vi "ESP_WIFI_mod2 (1).vi"() -> ()   [LabVIEW 2020]
uses:
  <vilib>/httpClient/LabVIEWHTTPClient.lvlib
panel:
  in  "ESP32 IP":string
  in  "stop":bool
  in  "Port":u16
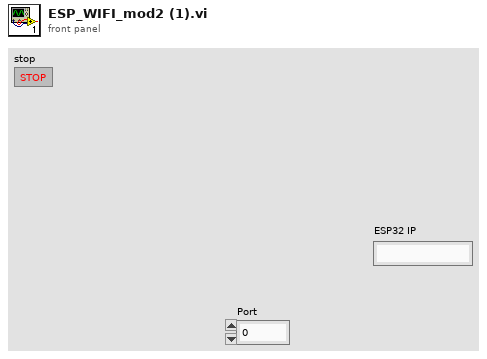
[diagram p1: front panel]
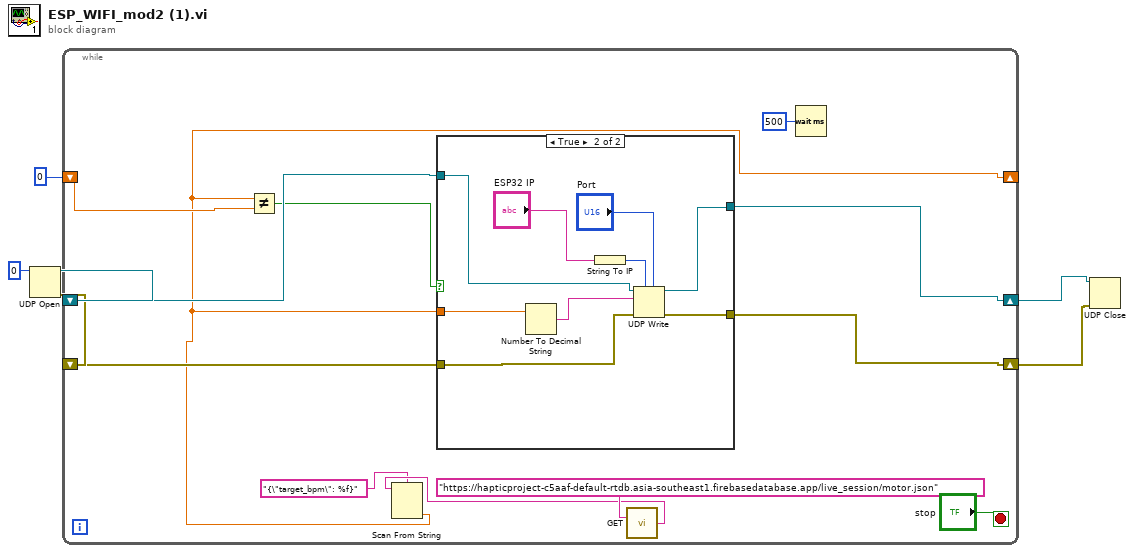
[diagram p0: block diagram]
diagram:
  n1 = UDP Open(11:u16 0 ("port")) -> (port=w6:refnum<k16>, 0:w5:errorcluster)  [unwired: 4 in, 1 out]
  n2 = while {
    shift-right: [w15] -> w4
    shift-left: w6 -> [w16]
    shift-right: [w13] -> w3
    shift-left: w5 -> [w14]
    shift-right: [w7] -> _
    shift-left: u16 0 ("port") -> [w9]
    stop <- "stop" stop-if-true
    n3 = call <vilib>:"GET.vi"("url"="https://hapticproject-c5aaf-default-rtdb.asia-southeast1.firebasedatabase.app/live_session/motor.json") -> ("body"=w11:string)  [unwired: 11 in, 3 out]
    n4 = Scan From String(format string="{\"target_bpm\": %f}" ("input string"), input string=w11) -> (output 1=w7:dbl)  [unwired: 3 in, 3 out]
    n5 = Not Equal?(x=w7, y=w9) -> (x != y?=w8:bool)
    n6 = case shown="True" w8 {
      tunnel: w16 -> [w20 w25]
      tunnel: [w20 w24] -> w15
      tunnel: w14 -> [w19 w23]
      tunnel: [w19 w22] -> w13
      tunnel: w7 -> [_ w21]
      frame False {
      }
      frame True {
        n7 = Number To Decimal String(number=w21) -> (decimal integer string=w29:string)  [unwired: 1 in]
        n8 = String To IP(1:"ESP32 IP") -> (0:w26:u32)
        n9 = UDP Write(address=w26, port or service name="Port", connection ID=w25, data in=w29, 8:w23) -> (error out=w22:errorcluster, 3:w24:refnum<k16>)  [unwired: 1 in]
      }
    }
    n10 = Wait (ms)(milliseconds to wait=u32 500) -> ()  [unwired: 1 out]
  }
  n11 = UDP Close(connection ID=w4, 8:w3) -> ()  [unwired: 2 out]
